vi "filenameincrementer.vi"(9 "string":string, 10 "pattern":string, 11 "Path":path=path "C:/Users/Bugra/Desktop/NNFinal/AcquisitonSetup/rs/Records") -> (1 "File Name":string, 2 "Operation":T1(ring), 3 "File Path":path)   [LabVIEW 2017]
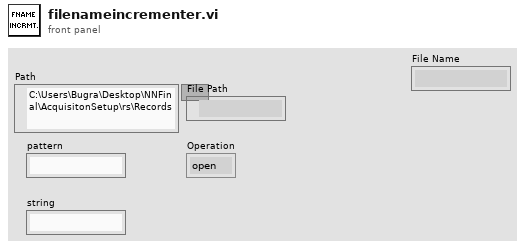
[diagram p1: front panel]
types:
  T1 = enum16{"open", "open or create", "create or replace", "create", "open (read-only)"}
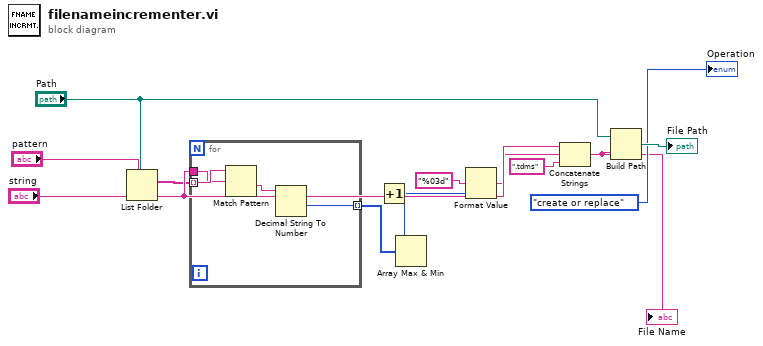
[diagram p0: block diagram]
diagram:
  n1 = List Folder(path="Path", pattern="pattern") -> (filenames=w8:string[])  [unwired: 2 in, 3 out]
  n2 = for {
    tunnel: w8 -> [w15] mode=indexing
    tunnel: "string" -> [w14]
    tunnel: [w17] -> w1 mode=indexing
    n3 = Match Pattern(string=w15, regular expression=w14) -> (after substring=w16:string)  [unwired: 1 in, 3 out]
    n4 = Decimal String To Number(string=w16) -> (number=w17:i32)  [unwired: 2 in, 1 out]
  }
  n5 = Array Max & Min(array=w1) -> (max value=w7:i32)  [unwired: 3 out]
  n6 = Increment(x=w7) -> (x+1=w6:i32)
  n7 = Format Value(format string="%03d", value (0)=w6) -> (output string=w4:string)  [unwired: 1 in]
  n8 = Concatenate Strings("string", w4, ".tdms" ("string")) -> (w2:string)
  "File Name" <- w2
  n9 = Build Path(base path="Path", name or relative path=w2) -> (appended path=→"File Path":path)
  "Operation" <- T1."create or replace" ("operation (0:open)")
